vi "incomingAgent.vi"(0 "MoAgSy_AgentBase in":refnum<class "MoAgSy_AgentBase.lvclass">, 2 "MoAgSy_Message":refnum<class "MoAgSy_Message.lvclass">, 5 "error in (no error)":errorcluster) -> (14 "MoAgSy_AgentBase out":refnum<class "MoAgSy_AgentBase.lvclass">, 19 "error out":errorcluster)   [LabVIEW 2009, in "MoAgSy_Base.lvlib" / "MoAgSy_AgentBase.lvclass"]
uses:
  MoAgSy_AgentBase.lvclass
  MoAgSy_Message/MoAgSy_Message.lvclass
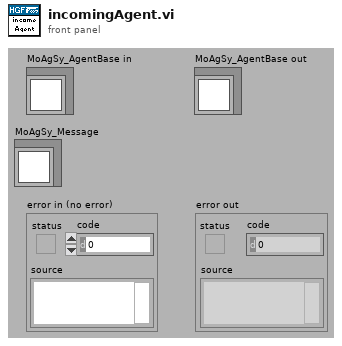
[diagram p1: front panel]
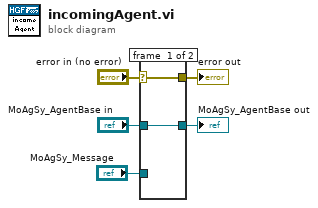
[diagram p0: block diagram]
diagram:
  n1 = case shown="No Error" "error in (no error)" {
    selector: "error in (no error)" -> [w6 w9]
    tunnel: [w6 w9] -> w4
    tunnel: [w7 w8] -> w2
    tunnel: "MoAgSy_AgentBase in" -> [w7 w8]
    tunnel: "MoAgSy_Message" -> [_ _]
    frame #0 {
    }
    frame #1 {
    }
  }
  "error out" <- w4
  "MoAgSy_AgentBase out" <- w2
